vi "Read Variant Cluster from Config File.vi"(5 "Index":i32, 7 "From Array?":bool, 8 "error in":errorcluster, 10 "Variant Cluster in":variant, 11 "Config Refnum in":T1) -> (0 "error out":errorcluster, 1 "Array Present":bool, 2 "Variant Cluster out":variant, 3 "Config Refnum out":T1)   [LabVIEW 2018, in "EMS Generic Actor.lvlib" / "EMS Generic.lvclass"]
doc: "This VI accepts either a Cluster or Array of Clusters that has been converted to a variant. The label of the cluster is used to define the section name and individual control names are used to define key names."
uses:
  EMS Generic.lvclass
  <vilib>/Utility/config.llb/Config Data RefNum.ctl
  <vilib>/Utility/config.llb/Read Key (String).vi
  <vilib>/Utility/config.llb/Read Key (Double).vi
  <vilib>/Utility/config.llb/Read Key (I32).vi
  <vilib>/Utility/config.llb/Read Key (U32).vi
  <vilib>/Utility/config.llb/Read Key (Path).vi
  <vilib>/Utility/Data Type/NI_Data Type.lvlib
  <vilib>/Utility/config.llb/NI_LVConfig.lvlib
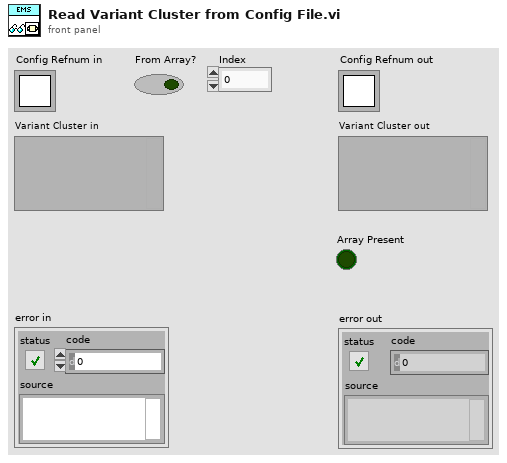
[diagram p1: front panel]
types:
  T1 = typedef "NI_LVConfig.lvlib/Config Data RefNum.ctl" = refnum<k1>
  T2 = typedef "NI_Data Type.lvlib/Data Type.ctl" = enum8{"Invalid Type", "Void", "I8", "I16", "I32", "I64", "U8", "U16", "U32", "U64", "Single Float", "Double Float", "Extended Float", "Single Complex", "Double Complex", "Extended Complex", "Enum U8", "Enum U16", "Enum U32", "Enum U64", "Single Float With Unit", "Double Float With Unit", "Extended Float With Unit", "Single Complex with Unit", "Double Complex with Unit", "Extended Complex with Unit", "Boolean", "String", "Path", "Picture", "Tag", "Array", "Cluster", "Variant", "LV Variant", "Waveform", "Timestamp", "Digital Waveform", "Digital Data", "ExpressData", "Refnum", "External Data", "VI", "Poly VI", "LabVIEW Class Instance", "Fixed Point"}
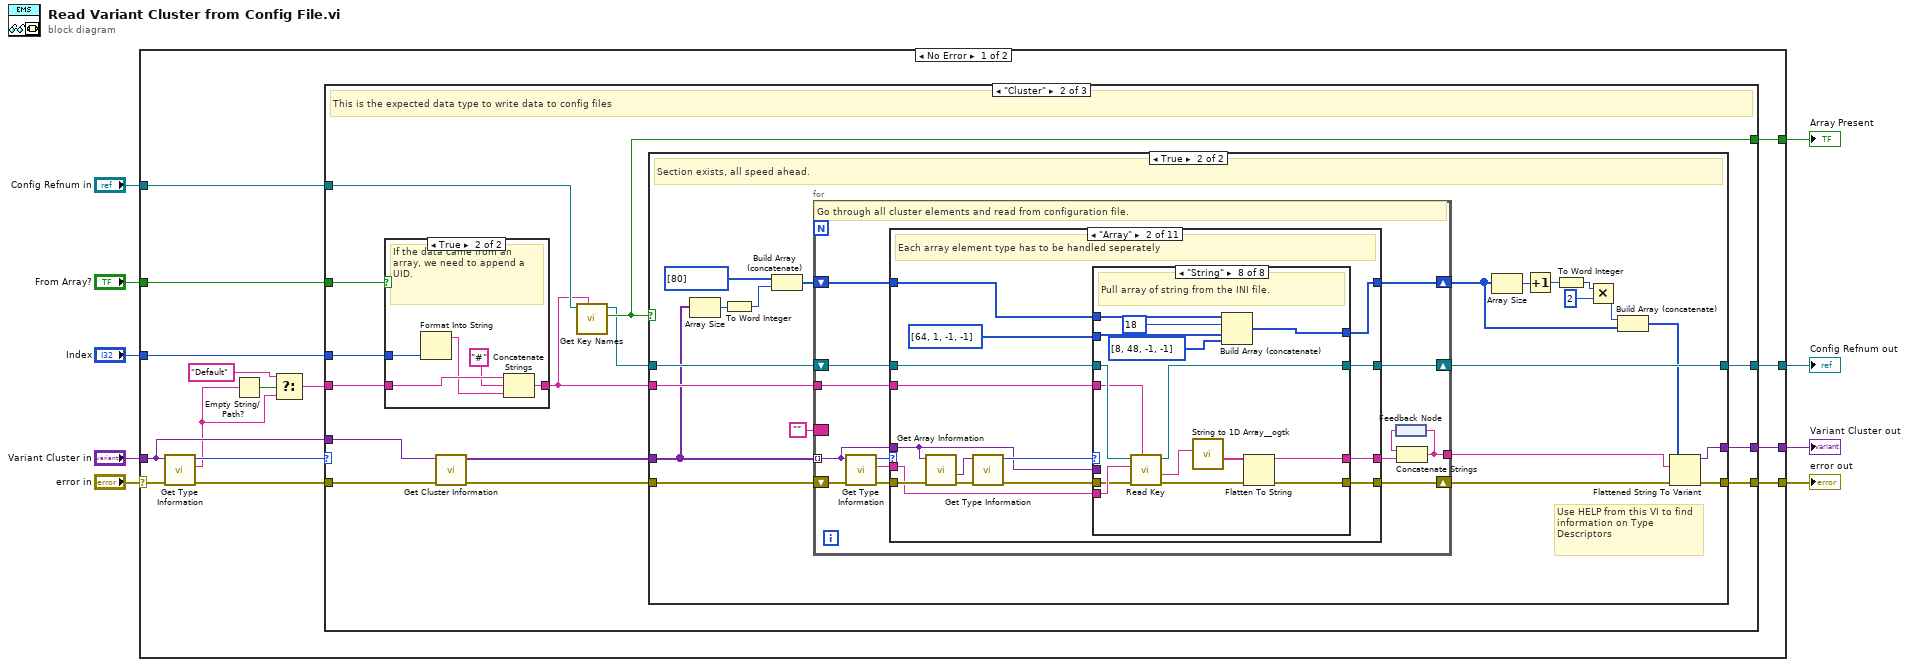
[diagram p0: block diagram]
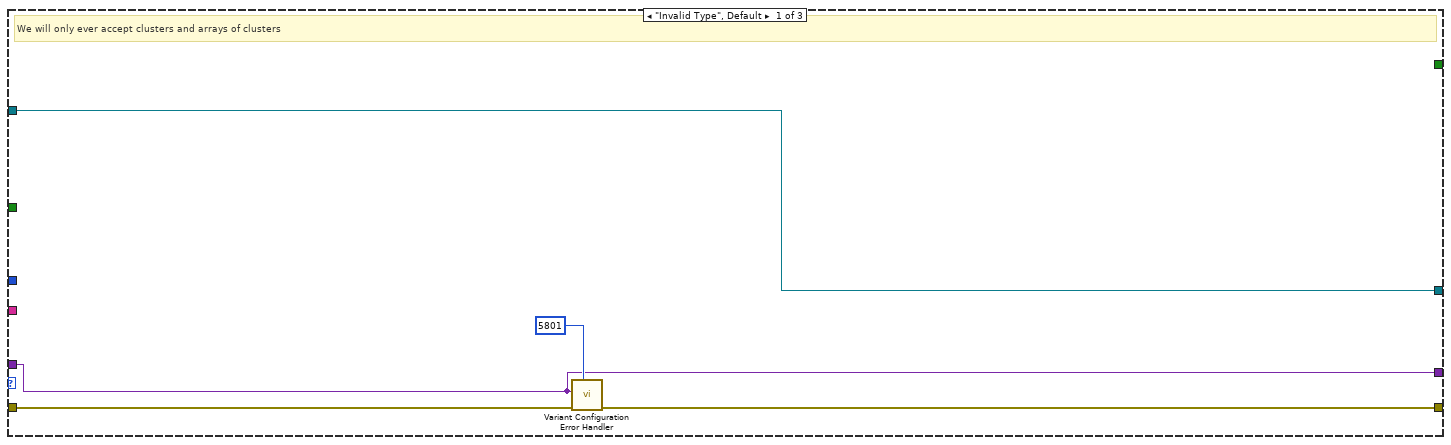
[diagram p2: hidden frame]
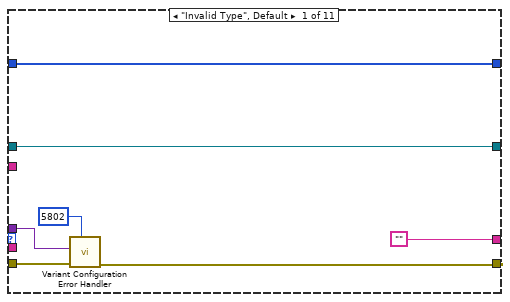
[diagram p4: hidden frame]
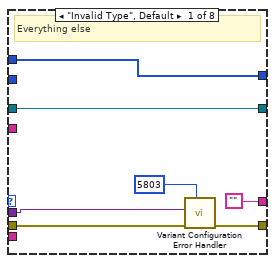
[diagram p5: hidden frame]
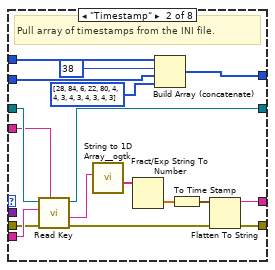
[diagram p6: hidden frame]
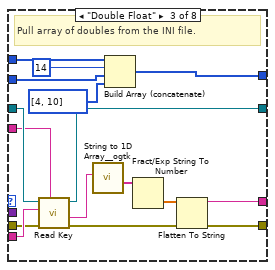
[diagram p7: hidden frame]
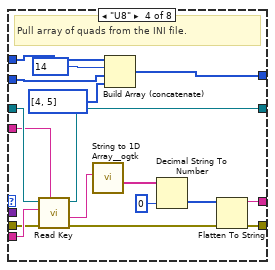
[diagram p8: hidden frame]
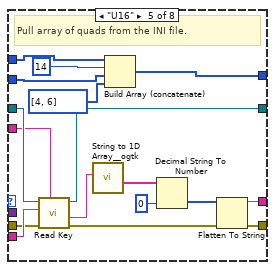
[diagram p9: hidden frame]
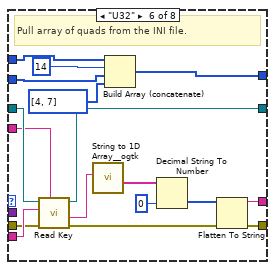
[diagram p10: hidden frame]
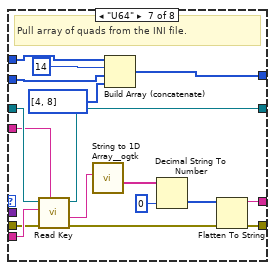
[diagram p11: hidden frame]
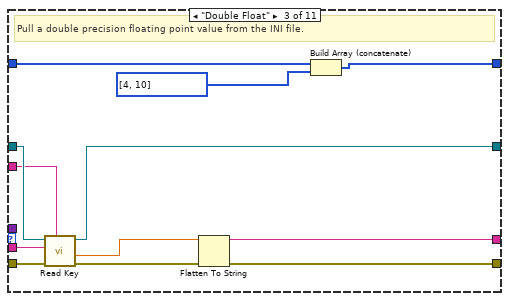
[diagram p12: hidden frame]
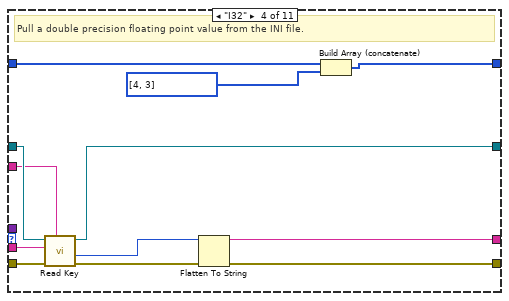
[diagram p13: hidden frame]
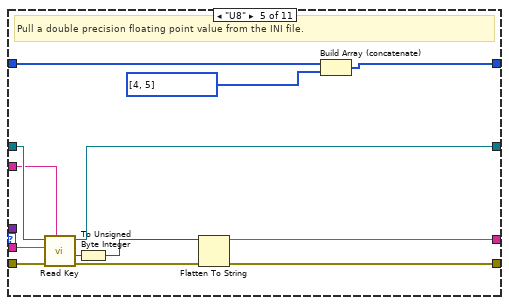
[diagram p14: hidden frame]
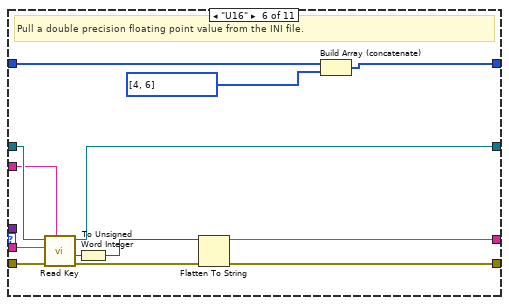
[diagram p15: hidden frame]
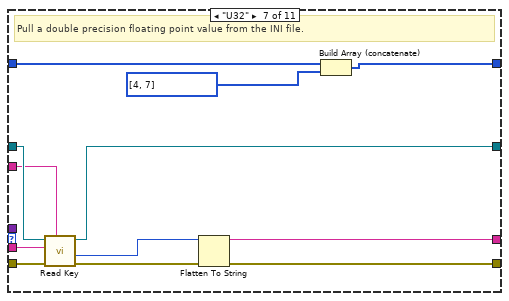
[diagram p16: hidden frame]
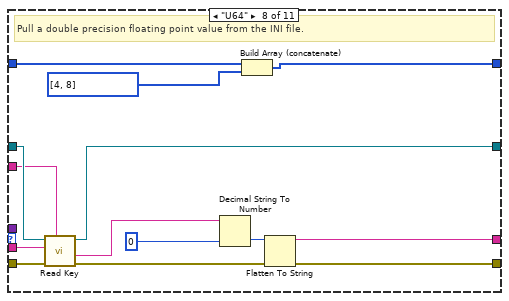
[diagram p17: hidden frame]
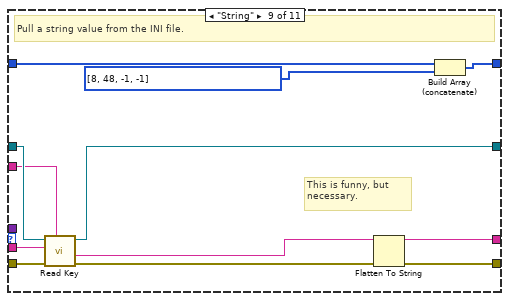
[diagram p18: hidden frame]
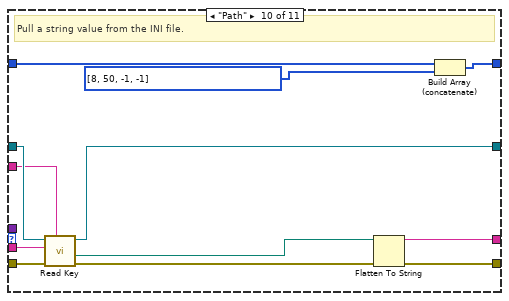
[diagram p19: hidden frame]
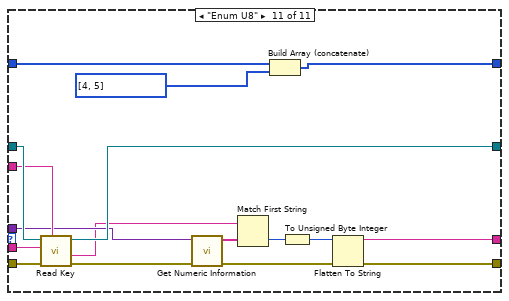
[diagram p20: hidden frame]
diagram:
  n1 = case shown="No Error" "error in" {
    selector: "error in" -> [w24 w367]
    tunnel: "Variant Cluster in" -> [w22 _]
    tunnel: "Config Refnum in" -> [w20 w368]
    tunnel: "Index" -> [w19 _]
    tunnel: "From Array?" -> [w18 _]
    tunnel: [w17 w368] -> w4
    tunnel: [w16 w367] -> w3
    tunnel: [w15 _] -> w2
    tunnel: [w14 _] -> w1
    frame No Error {
      n2 = call <vilib>:"Get Type Information.vi"("error in (no error)"=w24, "Variant"=w22) -> ("error out"=w21:errorcluster, "Name"=w10:string, "Type"=w23:T2)  [unwired: 5 in, 2 out]
      n3 = Empty String/Path?(string/path=w10) -> (empty?=w13:bool)
      n4 = Select(t="Default", s=w13, f=w10) -> (s? t:f=w11:string)
      n5 = case shown="\"Cluster\"" w23 {
        tunnel: w11 -> [_ w39 _]
        tunnel: w22 -> [w25 w37 w356]
        tunnel: w21 -> [w29 w43 w357]
        tunnel: [w28 w31 w355] -> w16
        tunnel: w20 -> [w26 w34 w354]
        tunnel: w19 -> [_ w38 _]
        tunnel: w18 -> [_ w40 _]
        tunnel: [w26 w32 w353] -> w17
        tunnel: [w25 w30 w349] -> w15
        tunnel: [_ w36 _] -> w14
        frame "Invalid Type", Default {
          # "We will only ever accept clusters and arrays of clusters"
          n6 = call "Variant Configuration Error Handler.vi"("Error Code"=5801 ("error code (0)"), "error in"=w29, "Variant"=w25) -> ("error out"=w28:errorcluster)  [unwired: 8 in]
        }
        frame "Cluster" {
          # "This is the expected data type to write data to config files"
          n7 = case shown="True" w40 {
            tunnel: w39 -> [w343 w347]
            tunnel: [w343 w344] -> w33
            tunnel: w38 -> [_ w348]
            frame False {
              # "Pass the name through as the section name."
            }
            frame True {
              # "If the data came from an array, we need to append a UID."
              n8 = Format Into String(w348) -> (resulting string=w345:string)  [unwired: 3 in, 1 out]
              n9 = Concatenate Strings(w347, "#" ("string"), w345) -> (w344:string)
            }
          }
          n10 = call <vilib>:"Get Cluster Information.vi"("error in (no error)"=w43, "Variant"=w37) -> ("error out"=w42:errorcluster, "Cluster Elements"=w41:variant[])  [unwired: 8 in]
          n11 = call <vilib>:"Get Key Names.vi"("section"=w33, "refnum"=w34) -> ("section exists?"=w36:bool, "refnum out"=w35:T1)  [unwired: 6 in, 2 out]
          n12 = case shown="True" w36 {
            tunnel: w42 -> [w44 w66]
            tunnel: [w44 w47] -> w31
            tunnel: w41 -> [_ w60]
            tunnel: w33 -> [_ w65]
            tunnel: [w45 w64] -> w32
            tunnel: w35 -> [w45 w63]
            tunnel: [_ w46] -> w30
            frame False {
              # "Sorry, section does not exist"
            }
            frame True {
              # "Use HELP from this VI to find information on Type Descriptors"
              # "Section exists, all speed ahead."
              n13 = Array Size(array=w60) -> (size(s)=w59:i32)
              n14 = To Word Integer(number=w59) -> (16bit integer=w57:i16)
              n15 = Build Array (concatenate)(i16[] [80] ("type string"), w57) -> (w58:i16[])
              n16 = for {
                shift-right: [w77] -> w50
                shift-left: w66 -> [w80]
                tunnel: w60 -> [w72] mode=indexing
                tunnel: w65 -> [w75]
                shift-right: [w73] -> w64
                shift-left: w63 -> [w76]
                border: "" -> [_]
                tunnel: [w69] -> w49
                shift-right: [w67] -> w48
                shift-left: w58 -> [w68]
                # "Go through all cluster elements and read from configuration file."
                n17 = call <vilib>:"Get Type Information.vi"("error in (no error)"=w80, "Variant"=w72) -> ("error out"=w78:errorcluster, "Name"=w74:string, "Type"=w79:T2)  [unwired: 5 in, 2 out]
                n18 = case shown="\"Array\"" w79 {
                  tunnel: w78 -> [w86 w102 w233 w245 w258 w271 w283 w297 w309 w321 w337]
                  tunnel: [w85 w95 w231 w243 w256 w269 w281 w295 w304 w316 w330] -> w77
                  tunnel: w76 -> [w84 w97 w237 w249 w262 w275 w287 w301 w313 w325 w342]
                  tunnel: w75 -> [_ w96 w236 w248 w261 w274 w286 w300 w312 w324 w341]
                  tunnel: w74 -> [_ w94 w235 w247 w260 w273 w285 w299 w311 w323 w340]
                  tunnel: [w84 w93 w234 w246 w259 w272 w284 w298 w310 w322 w339] -> w73
                  tunnel: ["" w92 w229 w242 w254 w267 w280 w294 w302 w314 w329] -> w71
                  tunnel: w72 -> [w83 w91 _ _ _ _ _ _ _ _ w338]
                  tunnel: w68 -> [w81 w89 w227 w239 w251 w264 w277 w290 w308 w320 w327]
                  tunnel: [w81 w90 w226 w238 w250 w263 w276 w288 w307 w319 w326] -> w67
                  frame "Invalid Type", Default {
                    n19 = call "Variant Configuration Error Handler.vi"("Error Code"=5802 ("error code (0)"), "error in"=w86, "Variant"=w83) -> ("error out"=w85:errorcluster)  [unwired: 8 in]
                  }
                  frame "Array" {
                    # "Each array element type has to be handled seperately"
                    n20 = call <vilib>:"Get Array Information.vi"("error in (no error)"=w102, "Variant"=w91) -> ("error out"=w100:errorcluster, "Array Element Data Type"=w99:variant)  [unwired: 6 in, 2 out]
                    n21 = call <vilib>:"Get Type Information.vi"("error in (no error)"=w100, "Variant"=w99) -> ("error out"=w98:errorcluster, "Type"=w101:T2)  [unwired: 5 in, 3 out]
                    n22 = case shown="\"String\"" w101 {
                      tunnel: w98 -> [w108 w122 w138 w155 w172 w189 w206 w221]
                      tunnel: w97 -> [w106 w126 w142 w159 w176 w193 w210 w225]
                      tunnel: w96 -> [_ w125 w141 w158 w175 w192 w209 w224]
                      tunnel: [w107 w116 w134 w151 w168 w185 w202 w217] -> w95
                      tunnel: w94 -> [_ w124 w140 w157 w174 w191 w208 w223]
                      tunnel: [w106 w123 w139 w156 w173 w190 w207 w222] -> w93
                      tunnel: ["" w115 w133 w150 w167 w184 w201 w216] -> w92
                      tunnel: w91 -> [w105 _ _ _ _ _ _ _]
                      tunnel: w89 -> [w103 w112 w129 w146 w163 w180 w197 w212]
                      tunnel: [w103 w113 w130 w147 w164 w181 w198 w213] -> w90
                      tunnel: i16[] [64, 1, -1, -1] ("type string") -> [_ w110 w127 w144 w161 w178 w195 w211]
                      frame "Invalid Type", Default {
                        # "Everything else"
                        n23 = call "Variant Configuration Error Handler.vi"("Error Code"=5803 ("error code (0)"), "error in"=w108, "Variant"=w105) -> ("error out"=w107:errorcluster)  [unwired: 8 in]
                      }
                      frame "Timestamp" {
                        # "Pull array of timestamps from the INI file."
                        n24 = call-poly <vilib>:"Read Key.vi"("section"=w125, "error in (no error)"=w122, "key"=w124, "refnum"=w126) -> ("error out"=w117:errorcluster, "value"=w121:string, "refnum out"=w123:T1)  [unwired: 4 in, 1 out]
                        n25 = call <userlib>:"String to 1D Array__ogtk.vi"("string"=w121) -> ("Array of Strings"=w120:string[])  [unwired: 10 in]
                        n26 = Fract/Exp String To Number(string=w120) -> (number=w119:dbl[])  [unwired: 3 in, 1 out]
                        n27 = Build Array (concatenate)(w112, i16 38, w110, i16[] [28, 84, 6, 22, 80, 4, 4, 3, 4, 3, 4, 3, 4, 3] ("type string")) -> (w113:i16[])
                        n28 = To Time Stamp(1:w119) -> (0:w118:timestamp[])
                        n29 = Flatten To String(anything=w118, error in (no error)=w117) -> (data string=w115:string, error out=w116:errorcluster)  [unwired: 2 in, 1 out]
                      }
                      frame "Double Float" {
                        # "Pull array of doubles from the INI file."
                        n30 = call-poly <vilib>:"Read Key.vi"("section"=w141, "error in (no error)"=w138, "key"=w140, "refnum"=w142) -> ("error out"=w135:errorcluster, "value"=w137:string, "refnum out"=w139:T1)  [unwired: 4 in, 1 out]
                        n31 = call <userlib>:"String to 1D Array__ogtk.vi"("string"=w137) -> ("Array of Strings"=w136:string[])  [unwired: 10 in]
                        n32 = Build Array (concatenate)(w129, i16 14, w127, i16[] [4, 10] ("type string")) -> (w130:i16[])
                        n33 = Fract/Exp String To Number(string=w136) -> (number=w132:dbl[])  [unwired: 3 in, 1 out]
                        n34 = Flatten To String(anything=w132, error in (no error)=w135) -> (data string=w133:string, error out=w134:errorcluster)  [unwired: 2 in, 1 out]
                      }
                      frame "U8" {
                        # "Pull array of quads from the INI file."
                        n35 = call-poly <vilib>:"Read Key.vi"("section"=w158, "error in (no error)"=w155, "key"=w157, "refnum"=w159) -> ("error out"=w152:errorcluster, "value"=w154:string, "refnum out"=w156:T1)  [unwired: 4 in, 1 out]
                        n36 = call <userlib>:"String to 1D Array__ogtk.vi"("string"=w154) -> ("Array of Strings"=w153:string[])  [unwired: 10 in]
                        n37 = Build Array (concatenate)(w146, i16 14, w144, i16[] [4, 5] ("type string")) -> (w147:i16[])
                        n38 = Decimal String To Number(string=w153, default (0L)=u8 0 ("default (0 I32)")) -> (number=w149:u8[])  [unwired: 1 in, 1 out]
                        n39 = Flatten To String(anything=w149, error in (no error)=w152) -> (data string=w150:string, error out=w151:errorcluster)  [unwired: 2 in, 1 out]
                      }
                      frame "U16" {
                        # "Pull array of quads from the INI file."
                        n40 = call-poly <vilib>:"Read Key.vi"("section"=w175, "error in (no error)"=w172, "key"=w174, "refnum"=w176) -> ("error out"=w169:errorcluster, "value"=w171:string, "refnum out"=w173:T1)  [unwired: 4 in, 1 out]
                        n41 = call <userlib>:"String to 1D Array__ogtk.vi"("string"=w171) -> ("Array of Strings"=w170:string[])  [unwired: 10 in]
                        n42 = Build Array (concatenate)(w163, i16 14, w161, i16[] [4, 6] ("type string")) -> (w164:i16[])
                        n43 = Decimal String To Number(string=w170, default (0L)=u16 0 ("default (0 I32)")) -> (number=w166:u16[])  [unwired: 1 in, 1 out]
                        n44 = Flatten To String(anything=w166, error in (no error)=w169) -> (data string=w167:string, error out=w168:errorcluster)  [unwired: 2 in, 1 out]
                      }
                      frame "U32" {
                        # "Pull array of quads from the INI file."
                        n45 = call-poly <vilib>:"Read Key.vi"("section"=w192, "error in (no error)"=w189, "key"=w191, "refnum"=w193) -> ("error out"=w186:errorcluster, "value"=w188:string, "refnum out"=w190:T1)  [unwired: 4 in, 1 out]
                        n46 = call <userlib>:"String to 1D Array__ogtk.vi"("string"=w188) -> ("Array of Strings"=w187:string[])  [unwired: 10 in]
                        n47 = Build Array (concatenate)(w180, i16 14, w178, i16[] [4, 7] ("type string")) -> (w181:i16[])
                        n48 = Decimal String To Number(string=w187, default (0L)=u32 0 ("default (0 I32)")) -> (number=w183:u32[])  [unwired: 1 in, 1 out]
                        n49 = Flatten To String(anything=w183, error in (no error)=w186) -> (data string=w184:string, error out=w185:errorcluster)  [unwired: 2 in, 1 out]
                      }
                      frame "U64" {
                        # "Pull array of quads from the INI file."
                        n50 = call-poly <vilib>:"Read Key.vi"("section"=w209, "error in (no error)"=w206, "key"=w208, "refnum"=w210) -> ("error out"=w203:errorcluster, "value"=w205:string, "refnum out"=w207:T1)  [unwired: 4 in, 1 out]
                        n51 = call <userlib>:"String to 1D Array__ogtk.vi"("string"=w205) -> ("Array of Strings"=w204:string[])  [unwired: 10 in]
                        n52 = Build Array (concatenate)(w197, i16 14, w195, i16[] [4, 8] ("type string")) -> (w198:i16[])
                        n53 = Decimal String To Number(string=w204, default (0L)=u64 0 ("default (0 I32)")) -> (number=w200:u64[])  [unwired: 1 in, 1 out]
                        n54 = Flatten To String(anything=w200, error in (no error)=w203) -> (data string=w201:string, error out=w202:errorcluster)  [unwired: 2 in, 1 out]
                      }
                      frame "String" {
                        # "Pull array of string from the INI file."
                        n55 = call-poly <vilib>:"Read Key.vi"("section"=w224, "error in (no error)"=w221, "key"=w223, "refnum"=w225) -> ("error out"=w218:errorcluster, "value"=w220:string, "refnum out"=w222:T1)  [unwired: 4 in, 1 out]
                        n56 = call <userlib>:"String to 1D Array__ogtk.vi"("string"=w220) -> ("Array of Strings"=w219:string[])  [unwired: 10 in]
                        n57 = Build Array (concatenate)(w212, i16 18, w211, i16[] [8, 48, -1, -1] ("type string")) -> (w213:i16[])
                        n58 = Flatten To String(anything=w219, error in (no error)=w218) -> (data string=w216:string, error out=w217:errorcluster)  [unwired: 2 in, 1 out]
                      }
                    }
                  }
                  frame "Double Float" {
                    # "Pull a double precision floating point value from the INI file."
                    n59 = call-poly <vilib>:"Read Key.vi"("section"=w236, "error in (no error)"=w233, "key"=w235, "refnum"=w237) -> ("error out"=w232:errorcluster, "value"=w230:dbl, "refnum out"=w234:T1)  [unwired: 4 in, 1 out]
                    n60 = Flatten To String(anything=w230, error in (no error)=w232) -> (data string=w229:string, error out=w231:errorcluster)  [unwired: 2 in, 1 out]
                    n61 = Build Array (concatenate)(w227, i16[] [4, 10] ("type string")) -> (w226:i16[])
                  }
                  frame "I32" {
                    # "Pull a double precision floating point value from the INI file."
                    n62 = call-poly <vilib>:"Read Key.vi"("section"=w248, "error in (no error)"=w245, "key"=w247, "refnum"=w249) -> ("error out"=w244:errorcluster, "value"=w241:i32, "refnum out"=w246:T1)  [unwired: 4 in, 1 out]
                    n63 = Flatten To String(anything=w241, error in (no error)=w244) -> (data string=w242:string, error out=w243:errorcluster)  [unwired: 2 in, 1 out]
                    n64 = Build Array (concatenate)(w239, i16[] [4, 3] ("type string")) -> (w238:i16[])
                  }
                  frame "U8" {
                    # "Pull a double precision floating point value from the INI file."
                    n65 = call-poly <vilib>:"Read Key.vi"("section"=w261, "error in (no error)"=w258, "key"=w260, "refnum"=w262) -> ("error out"=w257:errorcluster, "value"=w255:u32, "refnum out"=w259:T1)  [unwired: 4 in, 1 out]
                    n66 = To Unsigned Byte Integer(number=w255) -> (unsigned 8bit integer=w253:u8)
                    n67 = Flatten To String(anything=w253, error in (no error)=w257) -> (data string=w254:string, error out=w256:errorcluster)  [unwired: 2 in, 1 out]
                    n68 = Build Array (concatenate)(w251, i16[] [4, 5] ("type string")) -> (w250:i16[])
                  }
                  frame "U16" {
                    # "Pull a double precision floating point value from the INI file."
                    n69 = call-poly <vilib>:"Read Key.vi"("section"=w274, "error in (no error)"=w271, "key"=w273, "refnum"=w275) -> ("error out"=w270:errorcluster, "value"=w268:u32, "refnum out"=w272:T1)  [unwired: 4 in, 1 out]
                    n70 = To Unsigned Word Integer(number=w268) -> (unsigned 16bit integer=w266:u16)
                    n71 = Flatten To String(anything=w266, error in (no error)=w270) -> (data string=w267:string, error out=w269:errorcluster)  [unwired: 2 in, 1 out]
                    n72 = Build Array (concatenate)(w264, i16[] [4, 6] ("type string")) -> (w263:i16[])
                  }
                  frame "U32" {
                    # "Pull a double precision floating point value from the INI file."
                    n73 = call-poly <vilib>:"Read Key.vi"("section"=w286, "error in (no error)"=w283, "key"=w285, "refnum"=w287) -> ("error out"=w282:errorcluster, "value"=w279:u32, "refnum out"=w284:T1)  [unwired: 4 in, 1 out]
                    n74 = Flatten To String(anything=w279, error in (no error)=w282) -> (data string=w280:string, error out=w281:errorcluster)  [unwired: 2 in, 1 out]
                    n75 = Build Array (concatenate)(w277, i16[] [4, 7] ("type string")) -> (w276:i16[])
                  }
                  frame "U64" {
                    # "Pull a double precision floating point value from the INI file."
                    n76 = call-poly <vilib>:"Read Key.vi"("section"=w300, "error in (no error)"=w297, "key"=w299, "refnum"=w301) -> ("error out"=w296:errorcluster, "value"=w293:string, "refnum out"=w298:T1)  [unwired: 4 in, 1 out]
                    n77 = Decimal String To Number(string=w293, default (0L)=u64 0 ("default (0 I32)")) -> (number=w291:u64)  [unwired: 1 in, 1 out]
                    n78 = Build Array (concatenate)(w290, i16[] [4, 8] ("type string")) -> (w288:i16[])
                    n79 = Flatten To String(anything=w291, error in (no error)=w296) -> (data string=w294:string, error out=w295:errorcluster)  [unwired: 2 in, 1 out]
                  }
                  frame "String" {
                    # "This is funny, but necessary."
                    # "Pull a string value from the INI file."
                    n80 = call-poly <vilib>:"Read Key.vi"("section"=w312, "error in (no error)"=w309, "key"=w311, "refnum"=w313) -> ("error out"=w305:errorcluster, "value"=w303:string, "refnum out"=w310:T1)  [unwired: 4 in, 1 out]
                    n81 = Flatten To String(anything=w303, error in (no error)=w305) -> (data string=w302:string, error out=w304:errorcluster)  [unwired: 2 in, 1 out]
                    n82 = Build Array (concatenate)(w308, i16[] [8, 48, -1, -1] ("type string")) -> (w307:i16[])
                  }
                  frame "Path" {
                    # "Pull a string value from the INI file."
                    n83 = call-poly <vilib>:"Read Key.vi"("section"=w324, "error in (no error)"=w321, "key"=w323, "refnum"=w325) -> ("error out"=w317:errorcluster, "value"=w315:path, "refnum out"=w322:T1)  [unwired: 4 in, 1 out]
                    n84 = Flatten To String(anything=w315, error in (no error)=w317) -> (data string=w314:string, error out=w316:errorcluster)  [unwired: 2 in, 1 out]
                    n85 = Build Array (concatenate)(w320, i16[] [8, 50, -1, -1] ("type string")) -> (w319:i16[])
                  }
                  frame "Enum U8" {
                    n86 = call-poly <vilib>:"Read Key.vi"("section"=w341, "error in (no error)"=w337, "key"=w340, "refnum"=w342) -> ("error out"=w336:errorcluster, "value"=w334:string, "refnum out"=w339:T1)  [unwired: 4 in, 1 out]
                    n87 = call <vilib>:"Get Numeric Information.vi"("error in (no error)"=w336, "Variant"=w338) -> ("error out"=w332:errorcluster, "Enum Names"=w335:string[])  [unwired: 6 in, 2 out]
                    n88 = Match First String(2:w335, 3:w334) -> (0:w333:i32)  [unwired: 1 out]
                    n89 = Build Array (concatenate)(w327, i16[] [4, 5] ("type string")) -> (w326:i16[])
                    n90 = To Unsigned Byte Integer(number=w333) -> (unsigned 8bit integer=w331:u8)
                    n91 = Flatten To String(anything=w331, error in (no error)=w332) -> (data string=w329:string, error out=w330:errorcluster)  [unwired: 2 in, 1 out]
                  }
                }
                n92 = feedback #1() -> (w70:string)
                n93 = Concatenate Strings(w70, w71) -> (w69:string)
                n94 = feedback-in #1(w69) -> ()
              }
              n95 = Array Size(array=w48) -> (size(s)=w51:i32)
              n96 = Increment(x=w51) -> (x+1=w56:i32)
              n97 = To Word Integer(number=w56) -> (16bit integer=w52:i16)
              n98 = Multiply(x=w52, y=i16 2) -> (x*y=w55:i16)
              n99 = Build Array (concatenate)(w55, w48) -> (w54:i16[])
              n100 = Flattened String To Variant(4:w50, 6:w49, 7:w54) -> (0:w47:errorcluster, 3:w46:variant)
            }
          }
        }
        frame "Array" {
          # "Converts single variant of array of clusters to array of variant clusters."
          # "If it's an array we call back into the code to handle each cluster individually."
          n101 = call <vilib>:"Get Array Information.vi"("error in (no error)"=w357, "Variant"=w356) -> ("error out"=w351:errorcluster, "Array Element Data Type"=w352:variant)  [unwired: 6 in, 2 out]
          n102 = while {
            shift-right: [w365] -> w355
            shift-left: w351 -> [w366]
            tunnel: w352 -> [w363]
            shift-right: [w360] -> w353
            shift-left: w354 -> [w364]
            tunnel: [w359] -> w350 mode=indexing if=w358
            i -> [w361]
            stop <- w358 continue-if-true
            # "Recursion is awful"
            n103 = call "Read Variant Cluster from Config File.vi"("Index"=w361, "From Array?"=TRUE, "error in"=w366, "Variant Cluster in"=w363, "Config Refnum in"=w364) -> ("error out"=w365:errorcluster, "Array Present"=w358:bool, "Variant Cluster out"=w359:variant, "Config Refnum out"=w360:T1)  [unwired: 3 in]
          }
          n104 = To Variant(anything=w350) -> (Variant=w349:variant)
        }
      }
    }
    frame Error {
    }
  }
  "error out" <- w3
  "Config Refnum out" <- w4
  "Variant Cluster out" <- w2
  "Array Present" <- w1
